vi "Manual Mode - Configure File.vi"   [LabVIEW 2014, in "Associated Power Technologies 8500 Series.lvlib"]
uses:
  <instrlib>/Associated Power Technologies 8500 Series/Associated Power Technologies 8500 Series.lvlib
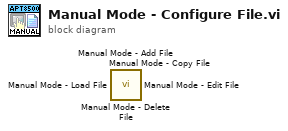
[diagram p0: block diagram]
diagram:
  n1 = call <instrlib>:"Manual Mode - Delete File.vi"() -> ()  [unwired: 10 in, 2 out]
  n2 = call <instrlib>:"Manual Mode - Copy File.vi"() -> ()  [unwired: 10 in, 2 out]
  n3 = call <instrlib>:"Manual Mode - Load File.vi"() -> ()  [unwired: 10 in, 2 out]
  n4 = call <instrlib>:"Manual Mode - Edit File.vi"() -> ()  [unwired: 10 in, 2 out]
  n5 = call <instrlib>:"Manual Mode - Add File.vi"() -> ()  [unwired: 10 in, 2 out]
